vi "AutoSetOpenCloseClaw.vi"(8 "error in (no error)":errorcluster, 11 "Open?":bool) -> (0 "error out":errorcluster)   [LabVIEW 2020]
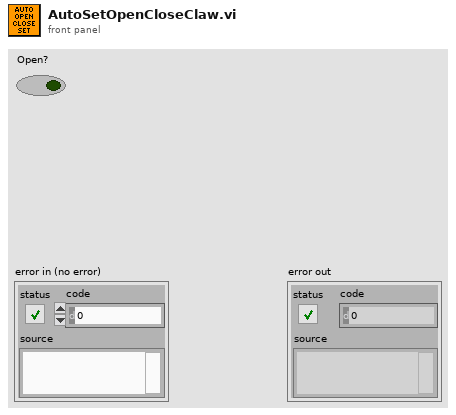
[diagram p1: front panel]
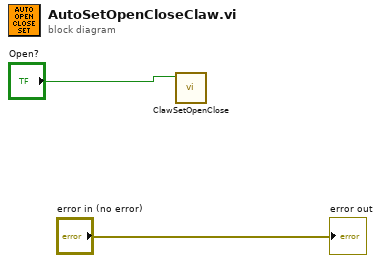
[diagram p0: block diagram]
diagram:
  n1 = call "ClawSetOpenClose.vi"("Open?"="Open?") -> ()  [unwired: 11 in]
  "error out" <- "error in (no error)"
